vi "SetTransparency(Polymorphic).vi"   [LabVIEW 2012]
doc: "Sets the transparency value (in %) of the VI from which a reference has been provided.\n\nFront panel transparency of 0% means opaque, while 100% is completely transparent."
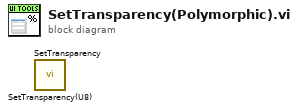
[diagram p0: block diagram]
diagram:
  n1 = call "SetTransparency(U8).vi"() -> ()  [unwired: 10 in, 2 out]
  n2 = call "SetTransparency.vi"() -> ()  [unwired: 10 in, 2 out]
